vi "I2C Read Data.vi"(5 "Address":T1 format="%02x", 6 "NoStop (F)":bool, 7 "I2C #":T2=-1, 8 "error in (no error)":errorcluster, 9 "Len":u8, 11 "Session in":refnum<class "Session.lvclass">) -> (0 "error out":errorcluster, 1 "Data":string, 3 "Session out":refnum<class "Session.lvclass">)   [LabVIEW 2024, in "CTI.lvlib" / "Session.lvclass"]
doc: "Reads data from an I2C bus from a peripheral with the specified I2C Address. <b>Len</b> determines the number of bytes to wait for. <b>NoStop</b> is useful for chaining multiple interactions with a peripheral together without allowing other I2C bus operations to occur."
uses:
  Session.lvclass
  I2C Number.ctl
  I2C Address.ctl
  DeviceComms/DeviceComms.lvclass
  CTI.lvlib
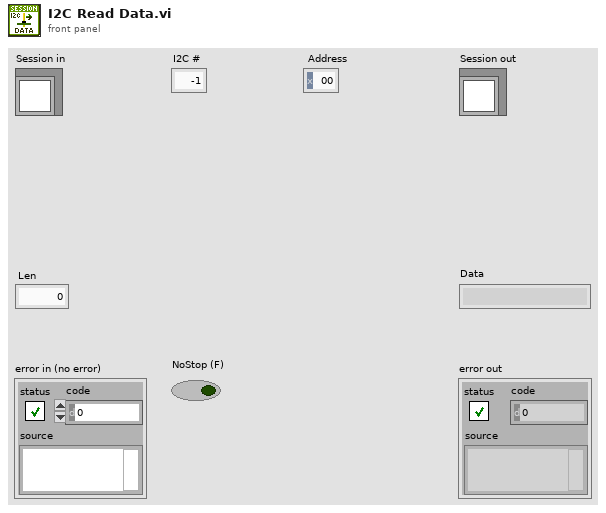
[diagram p1: front panel]
types:
  T1 = typedef "CTI.lvlib/I2C Address.ctl" = u8
  T2 = typedef "CTI.lvlib/I2C Number.ctl" = i8
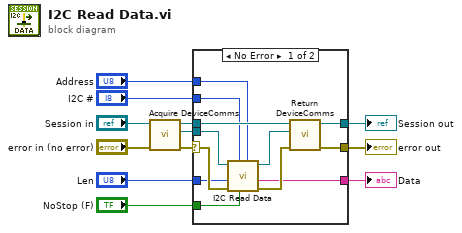
[diagram p0: block diagram]
diagram:
  n1 = call "Acquire DeviceComms.vi"("error in (no error)"="error in (no error)", "Session in"="Session in") -> ("error out"=w11:errorcluster, "DeviceComms"=w10:refnum<class "DeviceComms.lvclass">, "Session out"=w12:refnum<class "Session.lvclass">)  [unwired: 7 in]
  n2 = case shown="No Error" w11 {
    selector: w11 -> [w23 w26]
    tunnel: w12 -> [w22 w25]
    tunnel: w10 -> [w24 _]
    tunnel: [w19 w25] -> w2
    tunnel: [w18 w26] -> w1
    tunnel: "I2C #" -> [w17 _]
    tunnel: "Len" -> [w16 _]
    tunnel: "Address" -> [w15 _]
    tunnel: "NoStop (F)" -> [w14 _]
    tunnel: [w13 _] -> w3
    frame No Error {
      n3 = call-dynamic "I2C Read Data.vi"("Address"=w15, "NoStop (F)"=w14, "I2C #"=w17, "error in (no error)"=w23, "Len"=w16, "DeviceComms in"=w24) -> ("error out"=w20:errorcluster, "Data"=w13:string, "DeviceComms out"=w21:refnum<class "DeviceComms.lvclass">)  [unwired: 3 in]
      n4 = call "Return DeviceComms.vi"("error in (no error)"=w20, "DeviceComms"=w21, "Session in"=w22) -> ("error out"=w18:errorcluster, "Session out"=w19:refnum<class "Session.lvclass">)  [unwired: 7 in]
    }
    frame Error {
    }
  }
  "error out" <- w1
  "Session out" <- w2
  "Data" <- w3
